vi "Dibuix_ocell.vi"(11 "Posició Y":dbl) -> (3 "Dibuix pistola":cluster{dbl[], dbl[]}={[0.0, 0.0, 0.0, 0.02, 0.02, 0.02, 0.04, 0.04, 0.06, -0.06, -0.04, -0.04, -0.02, -0.02, -0.02], [-2.0, 0.0, -1.0, 0.0, 1.0, -1.0, 1.0, 2.0, 2.0, 2.0, 2.0, 1.0, 1.0, -1.0, 0.0]})   [LabVIEW 2020]
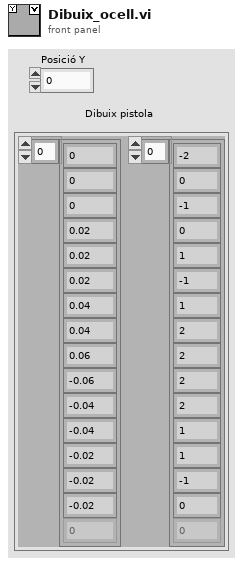
[diagram p1: front panel]
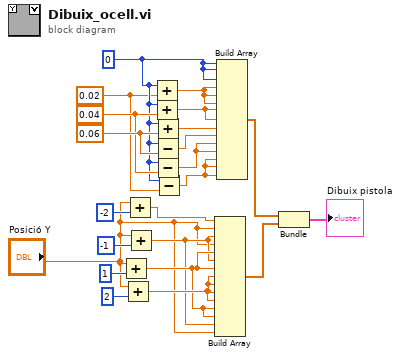
[diagram p0: block diagram]
diagram:
  w11 = 0.06 ("y")
  w9 = 0.04 ("y")
  w6 = 0.02 ("y")
  w7 = 0
  n1 = Add(x="Posició Y", y=1) -> (x+y=w4:dbl)
  n2 = Add(x="Posició Y", y=2) -> (x+y=w12:dbl)
  n3 = Add(x="Posició Y", y=-2) -> (x+y=w16:dbl)
  n4 = Add(x="Posició Y", y=-1) -> (x+y=w3:dbl)
  n5 = Add(x=w7, y=w6) -> (x+y=w19:dbl)
  n6 = Add(x=w7, y=w9) -> (x+y=w15:dbl)
  n7 = Add(x=w7, y=w11) -> (x+y=w13:dbl)
  n8 = Subtract(x=w7, y=w11) -> (x-y=w10:dbl)
  n9 = Subtract(x=w7, y=w9) -> (x-y=w8:dbl)
  n10 = Subtract(x=w7, y=w6) -> (x-y=w5:dbl)
  n11 = Build Array(w16, "Posició Y", w3, "Posició Y", w4, w3, w4, w12, w12, w12, w12, w4, w4, w3, "Posició Y") -> (w21:dbl[])
  n12 = Build Array(w7, w7, w7, w19, w19, w19, w15, w15, w13, w10, w8, w8, w5, w5, w5) -> (w22:dbl[])
  n13 = Bundle(w22, w21) -> (→"Dibuix pistola":cluster{dbl[], dbl[]})  [unwired: 1 in]
